vi "unique-name-differnetowner-test.vi"(8 "error in (no error)":errorcluster) -> (0 "error out":errorcluster)   [LabVIEW 2021]
uses:
  <vilib>/addons/_JKI Toolkits/Caraya/classes/Test/Test.lvclass
  src/SMO/SMO.lvclass
  <vilib>/addons/_JKI Toolkits/Caraya/classes/Assert/Assert.lvclass
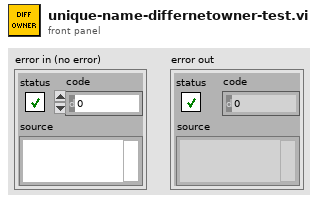
[diagram p1: front panel]
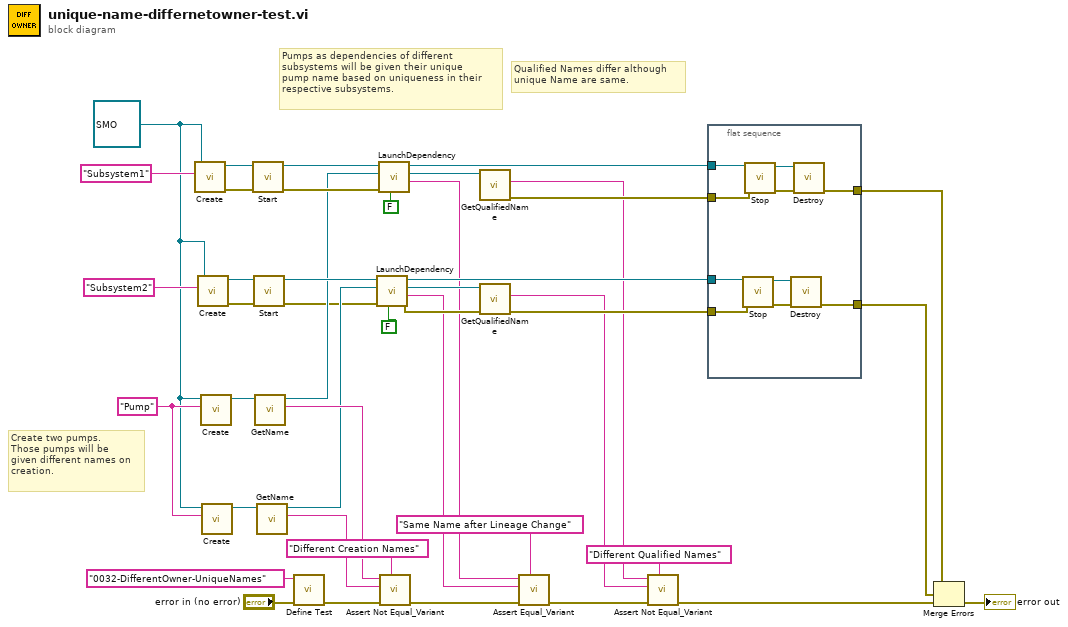
[diagram p0: block diagram]
diagram:
  w1 = refnum<class "SMO.lvclass"> refnum ("Dependency Type")
  w2 = "Pump" ("Subsystem Name (optional)")
  # "Qualified Names differ although\nunique Name are same."
  # "Pumps as dependencies of different\nsubsystems will be given their unique\npump name based on uniqueness in their\nrespective subsystems."
  # "Create two pumps.\nThose pumps will be\ngiven different names on\ncreation."
  n1 = call "Create.vi"("Subsystem Name (optional)"="Subsystem1", "SMO"=w1) -> ("error out"=w38:errorcluster, "SMO out"=w39:refnum<class "SMO.lvclass">)  [unwired: 7 in, 1 out]
  n2 = call "Create.vi"("Subsystem Name (optional)"="Subsystem2", "SMO"=w1) -> ("error out"=w37:errorcluster, "SMO out"=w36:refnum<class "SMO.lvclass">)  [unwired: 7 in, 1 out]
  n3 = call "Create.vi"("Subsystem Name (optional)"=w2, "SMO"=w1) -> ("SMO out"=w9:refnum<class "SMO.lvclass">)  [unwired: 7 in, 2 out]
  n4 = call "Create.vi"("Subsystem Name (optional)"=w2, "SMO"=w1) -> ("SMO out"=w6:refnum<class "SMO.lvclass">)  [unwired: 7 in, 2 out]
  n5 = call "Start.vi"("error in (no error)"=w38, "SMO"=w39) -> ("error out"=w34:errorcluster, "SMO out"=w35:refnum<class "SMO.lvclass">)  [unwired: 8 in]
  n6 = call "Start.vi"("error in (no error)"=w37, "SMO"=w36) -> ("error out"=w3:errorcluster, "SMO out"=w33:refnum<class "SMO.lvclass">)  [unwired: 8 in]
  n7 = call "GetName.vi"("SMO"=w9) -> ("Name"=w7:string, "SMO out"=w8:refnum<class "SMO.lvclass">)  [unwired: 7 in, 2 out]
  n8 = call "GetName.vi"("SMO"=w6) -> ("Name"=w4:string, "SMO out"=w5:refnum<class "SMO.lvclass">)  [unwired: 7 in, 2 out]
  n9 = call <vilib>:"Define Test.vi"("error in (no error)"="error in (no error)", "Label (VI Title)"="0032-DifferentOwner-UniqueNames") -> ("error out"=w12:errorcluster)  [unwired: 9 in]
  n10 = call "LaunchDependency.vi"("Shared Resource"=FALSE, "error in (no error)"=w3, "Dependency Type"=w5, "SMO in"=w33) -> ("error out"=w28:errorcluster, "Unique Name"=w20:string, "Dependency Reference"=w29:refnum<class "SMO.lvclass">, "SMO out"=w25:refnum<class "SMO.lvclass">)  [unwired: 4 in]
  n11 = call "LaunchDependency.vi"("Shared Resource"=FALSE, "error in (no error)"=w34, "Dependency Type"=w8, "SMO in"=w35) -> ("Unique Name"=w21:string, "Dependency Reference"=w30:refnum<class "SMO.lvclass">, "SMO out"=w27:refnum<class "SMO.lvclass">)  [unwired: 4 in, 1 out]
  n12 = call <vilib>:"Assert Not Equal_Variant.vi"("Label"="Different Creation Names", "error in (no error)"=w12, "Y"=w4, "X"=w7) -> ("error out"=w11:errorcluster)  [unwired: 7 in]
  n13 = call "GetQualifiedName.vi"("SMO"=w30) -> ("error out"=w26:errorcluster, "Qualified Name"=w15:string)  [unwired: 8 in, 1 out]
  n14 = call "GetQualifiedName.vi"("error in (no error)"=w28, "SMO"=w29) -> ("error out"=w24:errorcluster, "Qualified Name"=w14:string)  [unwired: 7 in, 1 out]
  n15 = call <vilib>:"Assert Equal_Variant.vi"("Label"="Same Name after Lineage Change", "error in (no error)"=w11, "Y"=w20, "X"=w21) -> ("error out"=w17:errorcluster)  [unwired: 7 in]
  n16 = call <vilib>:"Assert Not Equal_Variant.vi"("Label"="Different Qualified Names", "error in (no error)"=w17, "Y"=w14, "X"=w15) -> ("error out"=w16:errorcluster)  [unwired: 7 in]
  n17 = flat-sequence {
    tunnel: [w45] -> w23
    tunnel: [w44] -> w22
    tunnel: w27 -> [w53]
    tunnel: w26 -> [w52]
    tunnel: w25 -> [w51]
    tunnel: w24 -> [w50]
    frame #0 {
      n18 = call "Stop.vi"("error in (no error)"=w50, "SMO"=w51) -> ("error out"=w47:errorcluster, "SMO out"=w46:refnum<class "SMO.lvclass">)  [unwired: 8 in]
      n19 = call "Stop.vi"("error in (no error)"=w52, "SMO"=w53) -> ("error out"=w49:errorcluster, "SMO out"=w48:refnum<class "SMO.lvclass">)  [unwired: 8 in]
      n20 = call "Destroy.vi"("error in (no error)"=w47, "SMO"=w46) -> ("error out"=w44:errorcluster)  [unwired: 9 in]
      n21 = call "Destroy.vi"("error in (no error)"=w49, "SMO"=w48) -> ("error out"=w45:errorcluster)  [unwired: 9 in]
    }
  }
  n22 = Merge Errors(w23, w22, w16) -> (→"error out":errorcluster)
